vi "SVX Buffer Orbit Timebase Plot.vi"(0 "orbit/timebase plot in":T1(array[cluster]), 2 "reset? (F)":bool, 7 "buffer size (rev)":u32=1, 11 "error in (no error)":errorcluster) -> (4 "orbit/timebase plot out":T1(array[cluster]), 15 "error out":errorcluster)   [LabVIEW 2017, in "SoundVib_MCMDisplay.lvlib"]
doc: "Buffers orbit or timebase plot data and returns the buffered data. This VI requires continuous input data. The buffered data might have gaps between or overlap with previous buffers. Do not use the buffered data for limit testing or data logging."
uses:
  <vilib>/addons/Sound and Vibration/Order Analysis/Data Presentation/SoundVib_MCMDisplay.lvlib
  <vilib>/addons/Sound and Vibration/Order Analysis/Misc/SVMS Attribute.ctl
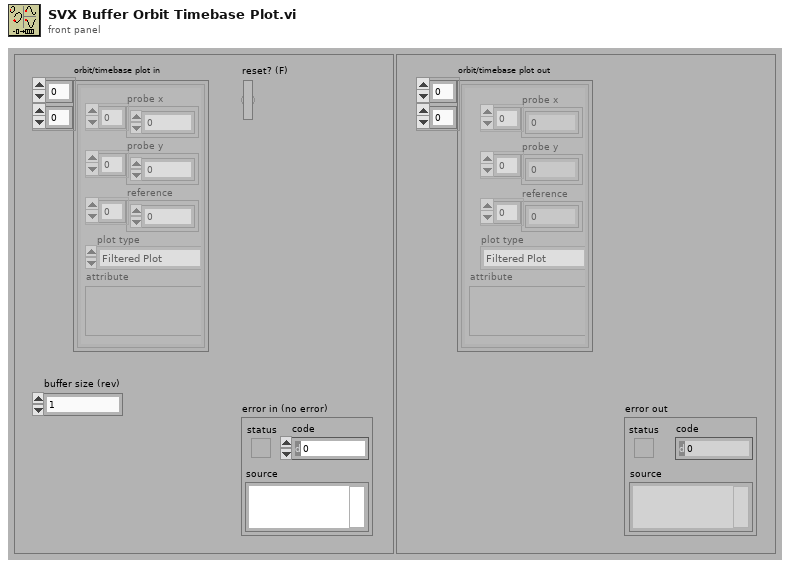
[diagram p1: front panel]
types:
  T1 = cluster{"probe x":dbl[], "probe y":dbl[], "reference":dbl[], "plot type":enum16{"Filtered Plot", "Unfiltered Plot"}, "attribute":variant}[][]
  T2 = typedef "SVMS Attribute.ctl" = u16
  T3 = cluster{"probe x":dbl[], "probe y":dbl[], "reference":dbl[], "plot type":enum16{"Filtered Plot", "Unfiltered Plot"}, "attribute":variant}[]
  T4 = cluster{"probe x":dbl[], "probe y":dbl[], "reference":dbl[], "plot type":enum16{"Filtered Plot", "Unfiltered Plot"}, "attribute":variant}
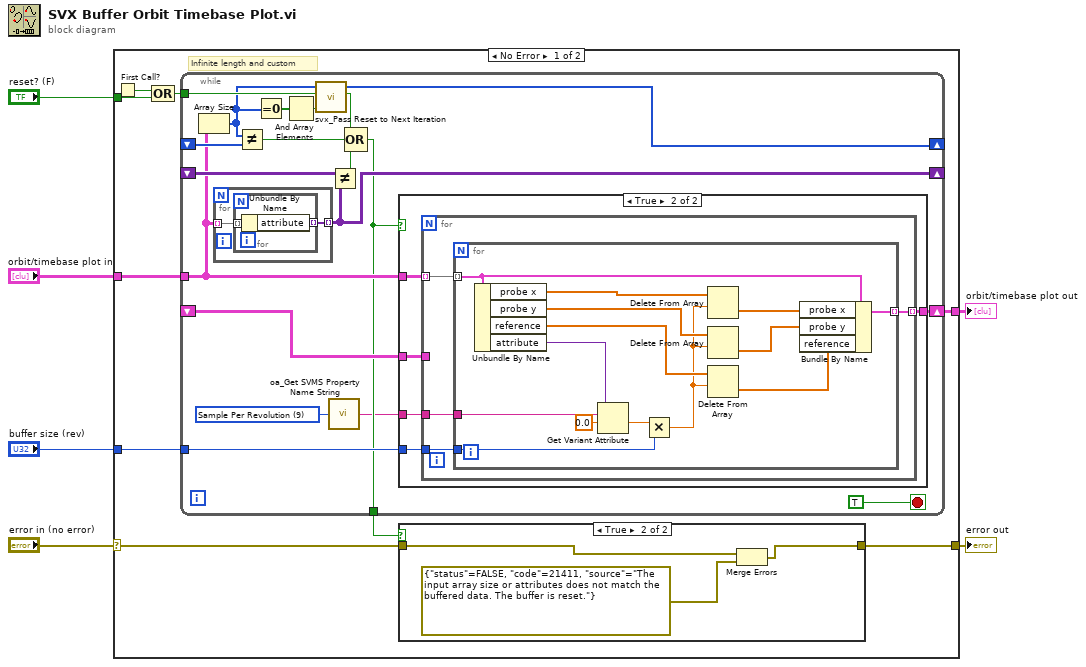
[diagram p0: block diagram]
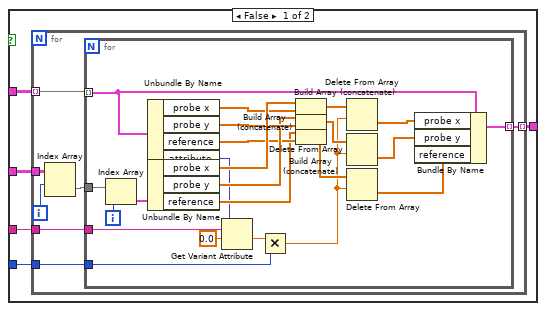
[diagram p3: hidden frame]
diagram:
  n1 = case shown="No Error" "error in (no error)" {
    selector: "error in (no error)" -> [w8 w100]
    tunnel: "reset? (F)" -> [w15 _]
    tunnel: "orbit/timebase plot in" -> [w13 _]
    tunnel: "buffer size (rev)" -> [w11 _]
    tunnel: [w7 w100] -> w3
    tunnel: [w10 _] -> w1
    frame No Error {
      # "Infinite length and custom"
      n2 = First Call?() -> (First Call?: T/F=w14:bool)
      n3 = Compound Arithmetic op=OR(w14, w15) -> (w12:bool)
      n4 = while {
        tunnel: w13 -> [w26]
        shift-right: [w31] -> _
        shift-left: _ -> [w32]
        shift-right: [w24] -> _
        shift-left: _ -> [w37]
        tunnel: w12 -> [w36]
        shift-right: [w29] -> w10
        shift-left: _ -> [w28]
        tunnel: w11 -> [w27]
        tunnel: [w22] -> w9
        stop <- TRUE stop-if-true
        w21 = T2 9 items=["Pulse / Revolution", "Slope", "Threshold", "Hysteresis", "Order", "Reference Label", "Rotation Direction", "Pair String", "Polar Plot Type", "Sample Per Revolution", "Probe Angle", "Probe Angle X", "Probe Angle Y", "X Axis Unit", "OTB Plot Type"] ("attribute")
        n5 = Array Size(array=w26) -> (size(s)=w24:i32[])
        n6 = for {
          tunnel: [w97] -> w31 mode=indexing
          tunnel: w26 -> [w96] mode=indexing
          n7 = for {
            tunnel: [w99] -> w97 mode=indexing
            tunnel: w96 -> [w98] mode=indexing
            n8 = Unbundle By Name(w98) -> ("attribute"=w99:variant)
          }
        }
        n9 = Not Equal?(x=w24, y=w37) -> (x != y?=w35:bool)
        n10 = Equal To 0?(x=w24) -> (x = 0?=w25:bool[])
        n11 = And Array Elements(Boolean array=w25) -> (logical AND=w23:bool)
        n12 = call <vilib>:"svx_Pass Reset to Next Iteration.vi"("trigger"=w23, "reset?(F)"=w36) -> ("reset out"=w34:bool)  [unwired: 9 in]
        n13 = call <vilib>:"oa_Get SVMS Property Name String.vi"("attribute"=w21) -> ("attribute name"=w20:string)  [unwired: 4 in]
        n14 = Not Equal?(x=w32, y=w31) -> (x != y?=w30:bool)
        n15 = Compound Arithmetic op=OR(w34, w35, w30) -> (w22:bool)
        n16 = case shown="True" w22 {
          tunnel: w26 -> [w42 w77]
          tunnel: [w41 w76] -> w29
          tunnel: w28 -> [w40 w75]
          tunnel: w27 -> [w39 w74]
          tunnel: w20 -> [w38 w73]
          frame False {
            n17 = for {
              tunnel: w42 -> [w49] mode=indexing
              tunnel: [w48] -> w41 mode=indexing
              tunnel: w40 -> [w46]
              tunnel: w39 -> [w47]
              tunnel: w38 -> [w43]
              i -> [w45]
              n18 = Index Array(array=w46, index (row)=w45) -> (element=w44:T3)  [unwired: 1 in]
              n19 = for {
                tunnel: w49 -> [w72] mode=indexing
                tunnel: [w71] -> w48 mode=indexing
                tunnel: w44 -> [w70]
                tunnel: w47 -> [w52]
                tunnel: w43 -> [w50]
                i -> [w56]
                n20 = Index Array(array=w70, index=w56) -> (element=w69:T4)
                n21 = Unbundle By Name(w72) -> ("probe x"=w67:dbl[], "probe y"=w66:dbl[], "reference"=w64:dbl[], "attribute"=w54:variant)
                n22 = Unbundle By Name(w69) -> ("probe x"=w68:dbl[], "probe y"=w65:dbl[], "reference"=w63:dbl[])
                n23 = Get Variant Attribute(Variant=w54, name=w50, default value (empty Variant)=0.0 ("pair")) -> (value=w53:dbl)  [unwired: 1 in, 3 out]
                n24 = Multiply(x=w53, y=w52) -> (x*y=w51:dbl)
                n25 = Build Array (concatenate)(w68, w67) -> (w62:dbl[])
                n26 = Build Array (concatenate)(w65, w66) -> (w61:dbl[])
                n27 = Build Array (concatenate)(w63, w64) -> (w58:dbl[])
                n28 = Delete From Array(array=w62, length=w51) -> (deleted portion=w60:dbl[])  [unwired: 1 in, 1 out]
                n29 = Delete From Array(array=w61, length=w51) -> (deleted portion=w59:dbl[])  [unwired: 1 in, 1 out]
                n30 = Delete From Array(array=w58, length=w51) -> (deleted portion=w57:dbl[])  [unwired: 1 in, 1 out]
                n31 = Bundle By Name(cluster=w72, "probe x"=w60, "probe y"=w59, "reference"=w57) -> (w71:T4)
              }
            }
          }
          frame True {
            n32 = for {
              tunnel: w77 -> [w81] mode=indexing
              tunnel: [w80] -> w76 mode=indexing
              tunnel: w75 -> [_]
              tunnel: w74 -> [w79]
              tunnel: w73 -> [w78]
              n33 = for {
                tunnel: w81 -> [w95] mode=indexing
                tunnel: [w94] -> w80 mode=indexing
                tunnel: w79 -> [w84]
                tunnel: w78 -> [w82]
                n34 = Unbundle By Name(w95) -> ("probe x"=w90:dbl[], "probe y"=w89:dbl[], "reference"=w88:dbl[], "attribute"=w85:variant)
                n35 = Get Variant Attribute(Variant=w85, name=w82, default value (empty Variant)=0.0 ("pair")) -> (value=w86:dbl)  [unwired: 1 in, 3 out]
                n36 = Multiply(x=w86, y=w84) -> (x*y=w83:dbl)
                n37 = Delete From Array(array=w90, length=w83) -> (deleted portion=w93:dbl[])  [unwired: 1 in, 1 out]
                n38 = Delete From Array(array=w89, length=w83) -> (deleted portion=w92:dbl[])  [unwired: 1 in, 1 out]
                n39 = Delete From Array(array=w88, length=w83) -> (deleted portion=w91:dbl[])  [unwired: 1 in, 1 out]
                n40 = Bundle By Name(cluster=w95, "probe x"=w93, "probe y"=w92, "reference"=w91) -> (w94:T4)
              }
            }
          }
        }
      }
      n41 = case shown="True" w9 {
        tunnel: w8 -> [w16 w19]
        tunnel: [w16 w18] -> w7
        frame False {
        }
        frame True {
          n42 = Merge Errors(w19, errorcluster {"status"=FALSE, "code"=21411, "source"="The input array size or attributes does not match the buffered data. The buffer is reset."} ("error in 2 (no error)")) -> (w18:errorcluster)
        }
      }
    }
    frame Error {
    }
  }
  "error out" <- w3
  "orbit/timebase plot out" <- w1
